vi "transfer table data.vi"(9 "transfer specification in":T1[](array[typedef]), 10 "data table source in":T3, 11 "data table sink in":T3) -> (1 "transfer specification out":T1[](array[typedef]), 2 "data table source out":T3, 3 "data table sink out":T3)   [LabVIEW 2013, in "data bus values.lvlib"]
doc: "Applies the data transfer between the source table and sink table, as defined by the transfer specification."
uses:
  data bus values.lvlib
  data table.ctl
  transfer specification.ctl
  tag/Data Type.ctl
  tag/data bus tag description.lvclass
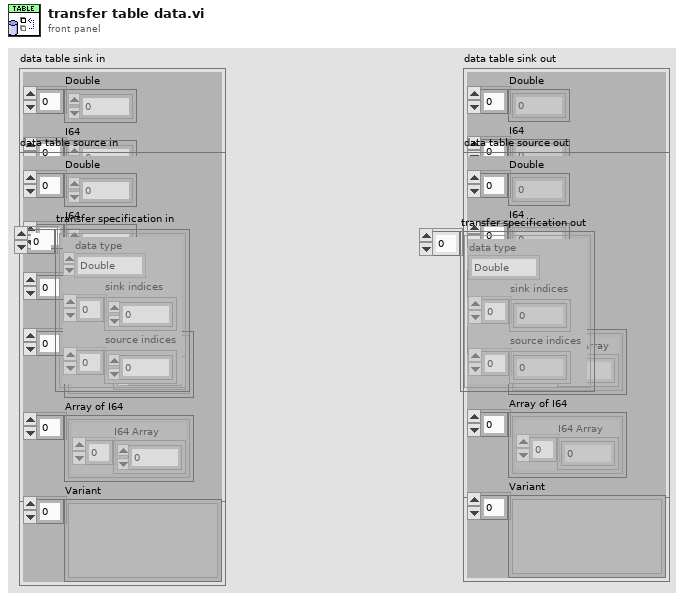
[diagram p1: front panel]
types:
  T1 = typedef "data bus values.lvlib/transfer specification.ctl" = cluster{"data type":T2, "sink indices":i32[], "source indices":i32[]}
  T2 = typedef "data bus tag description.lvclass/Data Type.ctl" = enum16{"Double", "I64", "Boolean", "Array of Double", "Array of I64", "Variant"}
  T3 = typedef "data bus values.lvlib/data table.ctl" = cluster{"Double":dbl[], "I64":i64[], "Boolean":bool[], "Array of Double":cluster{"DBL Array":dbl[]}[], "Array of I64":cluster{"I64 Array":i64[]}[], "Variant":variant[]}
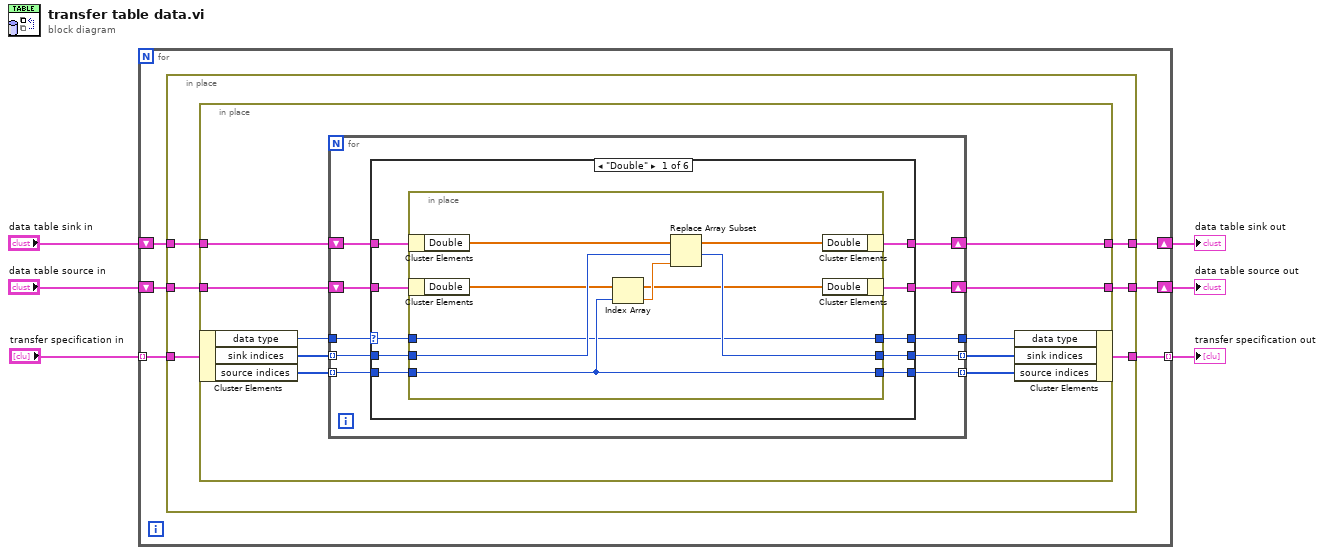
[diagram p0: block diagram]
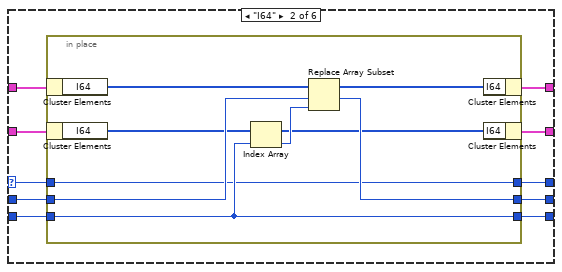
[diagram p2: hidden frame]
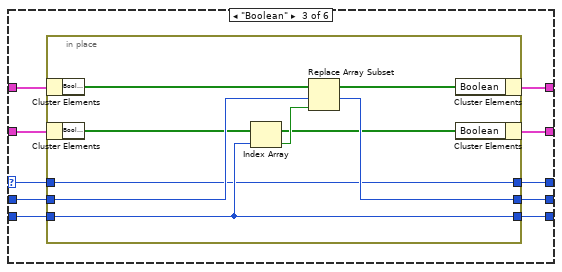
[diagram p3: hidden frame]
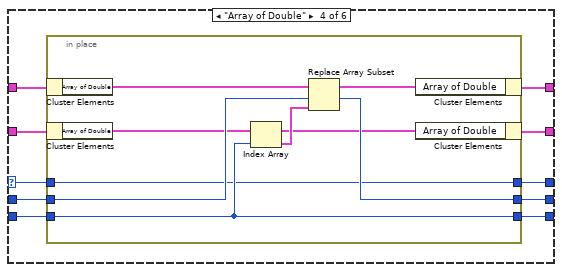
[diagram p4: hidden frame]
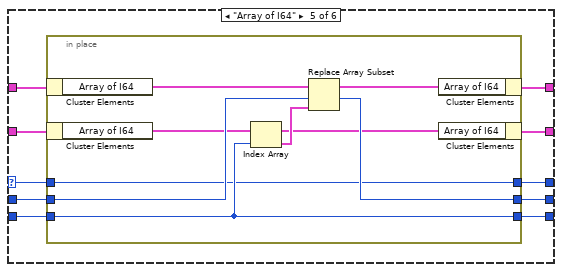
[diagram p5: hidden frame]
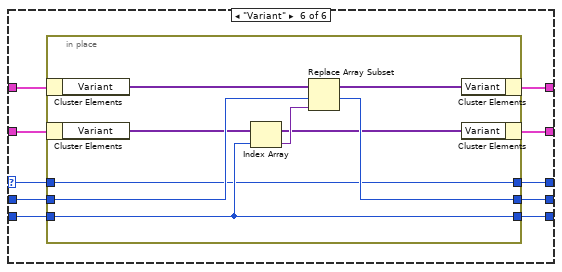
[diagram p6: hidden frame]
diagram:
  n1 = for {
    tunnel: "transfer specification in" -> [w8] mode=indexing
    shift-right: [w9] -> w2
    shift-left: "data table source in" -> [w10]
    shift-right: [w11] -> w3
    shift-left: "data table sink in" -> [w12]
    tunnel: [w7] -> w1 mode=indexing
    n2 = in-place {
      in-place-border: w12 -> [w18]
      in-place-border: [w17] -> w11
      in-place-border: w10 -> [w16]
      in-place-border: [w15] -> w9
      in-place-border: w8 -> [w14]
      in-place-border: [w13] -> w7
      n3 = in-place {
        in-place-border: w18 -> [w28]
        in-place-border: [w27] -> w17
        in-place-border: w16 -> [w26]
        in-place-border: [w25] -> w15
        n4 = in-place-cluster #1(w14) -> ("data type"=w24:T2, "sink indices"=w23:i32[], "source indices"=w22:i32[])
        n5 = for {
          shift-right: [w36] -> w27
          shift-left: w28 -> [w37]
          shift-right: [w35] -> w25
          shift-left: w26 -> [w34]
          tunnel: w24 -> [w38]
          tunnel: w23 -> [w33] mode=indexing
          tunnel: w22 -> [w32] mode=indexing
          tunnel: [w31] -> w21 mode=indexing
          tunnel: [w30] -> w20 mode=indexing
          tunnel: [w29] -> w19
          n6 = case shown="\"Double\"" w38 {
            selector: w38 -> [w40 w57 w74 w91 w108 w125]
            tunnel: w37 -> [w48 w65 w82 w99 w116 w133]
            tunnel: [w46 w63 w80 w97 w114 w131] -> w36
            tunnel: [w45 w62 w79 w96 w113 w130] -> w35
            tunnel: w34 -> [w47 w64 w81 w98 w115 w132]
            tunnel: w33 -> [w44 w61 w78 w95 w112 w129]
            tunnel: w32 -> [w43 w60 w77 w94 w111 w128]
            tunnel: [w42 w59 w76 w93 w110 w127] -> w31
            tunnel: [w41 w58 w75 w92 w109 w126] -> w30
            tunnel: [w39 w56 w73 w90 w107 w124] -> w29
            frame "Double" {
              n7 = in-place {
                in-place-border: w44 -> [w53]
                in-place-border: w43 -> [w52]
                in-place-border: [w53] -> w42
                in-place-border: [w52] -> w41
                in-place-border: w40 -> [w51]
                in-place-border: [w51] -> w39
                n8 = in-place-cluster #2(w48) -> ("Double"=w55:dbl[])
                n9 = in-place-cluster #3(w47) -> ("Double"=w49:dbl[])
                n10 = Index Array(array=w49, index=w52) -> (element=w50:dbl)
                n11 = Replace Array Subset(array=w55, new element=w50, index=w53) -> (w54:dbl[])
                n12 = in-place-cluster #2("Double"=w54) -> (w46:T3)
                n13 = in-place-cluster #3("Double"=w49) -> (w45:T3)
              }
            }
            frame "I64" {
              n14 = in-place {
                in-place-border: w61 -> [w70]
                in-place-border: w60 -> [w69]
                in-place-border: [w70] -> w59
                in-place-border: [w69] -> w58
                in-place-border: w57 -> [w68]
                in-place-border: [w68] -> w56
                n15 = in-place-cluster #4(w65) -> ("I64"=w72:i64[])
                n16 = in-place-cluster #5(w64) -> ("I64"=w66:i64[])
                n17 = Index Array(array=w66, index=w69) -> (element=w67:i64)
                n18 = Replace Array Subset(array=w72, new element=w67, index=w70) -> (w71:i64[])
                n19 = in-place-cluster #4("I64"=w71) -> (w63:T3)
                n20 = in-place-cluster #5("I64"=w66) -> (w62:T3)
              }
            }
            frame "Boolean" {
              n21 = in-place {
                in-place-border: w78 -> [w87]
                in-place-border: w77 -> [w86]
                in-place-border: [w87] -> w76
                in-place-border: [w86] -> w75
                in-place-border: w74 -> [w85]
                in-place-border: [w85] -> w73
                n22 = in-place-cluster #6(w82) -> ("Boolean"=w89:bool[])
                n23 = in-place-cluster #7(w81) -> ("Boolean"=w83:bool[])
                n24 = Index Array(array=w83, index=w86) -> (element=w84:bool)
                n25 = Replace Array Subset(array=w89, new element=w84, index=w87) -> (w88:bool[])
                n26 = in-place-cluster #6("Boolean"=w88) -> (w80:T3)
                n27 = in-place-cluster #7("Boolean"=w83) -> (w79:T3)
              }
            }
            frame "Array of Double" {
              n28 = in-place {
                in-place-border: w95 -> [w104]
                in-place-border: w94 -> [w103]
                in-place-border: [w104] -> w93
                in-place-border: [w103] -> w92
                in-place-border: w91 -> [w102]
                in-place-border: [w102] -> w90
                n29 = in-place-cluster #8(w99) -> ("Array of Double"=w106:cluster{"DBL Array":dbl[]}[])
                n30 = in-place-cluster #9(w98) -> ("Array of Double"=w100:cluster{"DBL Array":dbl[]}[])
                n31 = Index Array(array=w100, index=w103) -> (element=w101:cluster{"DBL Array":dbl[]})
                n32 = Replace Array Subset(array=w106, new element=w101, index=w104) -> (w105:cluster{"DBL Array":dbl[]}[])
                n33 = in-place-cluster #8("Array of Double"=w105) -> (w97:T3)
                n34 = in-place-cluster #9("Array of Double"=w100) -> (w96:T3)
              }
            }
            frame "Array of I64" {
              n35 = in-place {
                in-place-border: w112 -> [w121]
                in-place-border: w111 -> [w120]
                in-place-border: [w121] -> w110
                in-place-border: [w120] -> w109
                in-place-border: w108 -> [w119]
                in-place-border: [w119] -> w107
                n36 = in-place-cluster #10(w116) -> ("Array of I64"=w123:cluster{"I64 Array":i64[]}[])
                n37 = in-place-cluster #11(w115) -> ("Array of I64"=w117:cluster{"I64 Array":i64[]}[])
                n38 = Index Array(array=w117, index=w120) -> (element=w118:cluster{"I64 Array":i64[]})
                n39 = Replace Array Subset(array=w123, new element=w118, index=w121) -> (w122:cluster{"I64 Array":i64[]}[])
                n40 = in-place-cluster #10("Array of I64"=w122) -> (w114:T3)
                n41 = in-place-cluster #11("Array of I64"=w117) -> (w113:T3)
              }
            }
            frame "Variant" {
              n42 = in-place {
                in-place-border: w129 -> [w138]
                in-place-border: w128 -> [w137]
                in-place-border: [w138] -> w127
                in-place-border: [w137] -> w126
                in-place-border: w125 -> [w136]
                in-place-border: [w136] -> w124
                n43 = in-place-cluster #12(w133) -> ("Variant"=w140:variant[])
                n44 = in-place-cluster #13(w132) -> ("Variant"=w134:variant[])
                n45 = Index Array(array=w134, index=w137) -> (element=w135:variant)
                n46 = Replace Array Subset(array=w140, new element=w135, index=w138) -> (w139:variant[])
                n47 = in-place-cluster #12("Variant"=w139) -> (w131:T3)
                n48 = in-place-cluster #13("Variant"=w134) -> (w130:T3)
              }
            }
          }
        }
        n49 = in-place-cluster #1("data type"=w19, "sink indices"=w21, "source indices"=w20) -> (w13:T1)
      }
    }
  }
  "data table sink out" <- w3
  "data table source out" <- w2
  "transfer specification out" <- w1
